vi "ADIS16470 Read Multiple Registers.vi"(8 "error in (no error)":errorcluster, 10 "Registers":T3[](array[typedef]) items=["Reserved", "_Reserved", "DIAG_STAT", "_DIAG_STAT", "X_GYRO_LOW", "_X_GYRO_LOW", "X_GYRO_OUT", "_X_GYRO_OUT", "Y_GYRO_LOW", "_Y_GYRO_LOW", ""], 11 "SPIDevRefIn":T1) -> (0 "error out":errorcluster, 2 "Values":u16[](array[numeric]), 3 "SPIDevRefOut":T1)   [LabVIEW 2025]
uses:
  <vilib>/Rock Robotics/WPI/ThirdParty/ADI/ADIS16470/Typedef/ADIS16470 Register.ctl
  <vilib>/Rock Robotics/WPI/SPI/WPI_SPIDevRef.ctl
  <vilib>/Rock Robotics/SystemInterfaces/spilib/spi_bus.ctl
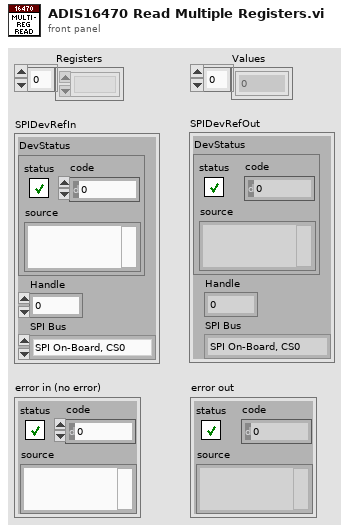
[diagram p1: front panel]
types:
  T1 = typedef "WPI_SPIDevRef.ctl" = cluster{"DevStatus":errorcluster, "Handle":i32, "SPI Bus":T2}
  T2 = typedef "spi_bus.ctl" = enum16{"SPI On-Board, CS0", "SPI On-Board, CS1", "SPI On-Board, CS2", "SPI On-Board, CS3", "SPI MXP", "Invalid"}
  T3 = typedef "ADIS16470 Register.ctl" = u8
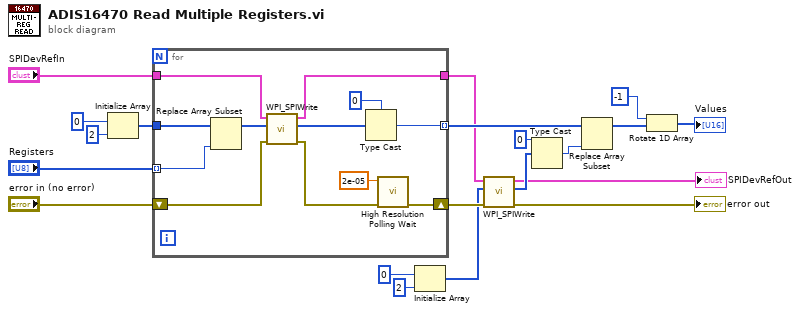
[diagram p0: block diagram]
diagram:
  n1 = Initialize Array(u8 0 ("element"), 2 ("dimension size")) -> (w13:u8[])
  n2 = for {
    tunnel: w13 -> [w28]
    tunnel: "Registers" -> [w29] mode=indexing
    tunnel: "SPIDevRefIn" -> [w22]
    shift-right: [w24] -> w7
    shift-left: "error in (no error)" -> [w27]
    tunnel: [w26] -> w10 mode=indexing
    tunnel: [w21] -> w8
    n3 = Replace Array Subset(array=w28, new element=w29) -> (w30:u8[])  [unwired: 1 in]
    n4 = call <vilib>:"WPI_SPIWrite.vi"("error in (no error)"=w27, "Data To Send"=w30, "SPIDevRef"=w22) -> ("error out"=w25:errorcluster, "Received Data"=w31:u8[], "SPIDevRef"=w21:T1)  [unwired: 6 out]
    n5 = Type Cast(type=u16 0, x=w31) -> (*(type *) &x=w26:u16)
    n6 = call <vilib>:"High Resolution Polling Wait.vi"("error in (no error)"=w25, "seconds to wait"=2e-05) -> ("error out"=w24:errorcluster)  [unwired: 9 in]
  }
  n7 = Initialize Array(u8 0 ("element"), 2 ("dimension size")) -> (w3:u8[])
  n8 = call <vilib>:"WPI_SPIWrite.vi"("error in (no error)"=w7, "Data To Send"=w3, "SPIDevRef"=w8) -> ("error out"=→"error out":errorcluster, "Received Data"=w2:u8[], "SPIDevRef"=→"SPIDevRefOut":T1)  [unwired: 6 out]
  n9 = Type Cast(type=u16 0, x=w2) -> (*(type *) &x=w17:u16)
  n10 = Replace Array Subset(array=w10, new element=w17) -> (w16:u16[])  [unwired: 1 in]
  n11 = Rotate 1D Array(1:w16, 2:-1 ("n")) -> (0:→"Values":u16[])
